vi "Client Monitor.vi"() -> ()   [LabVIEW 2020]
uses:
  source/Client/Subscription/Subscription.lvclass
  source/Value/Value/Value.lvclass
  source/Client/Client/Client.lvclass
  41e1d11c-de9d-40a4-9c04-0640dffbb6fa.vi
panel:
  in  "timeout":dbl[unit]=1.0
  out "Value":dbl
  out "timed out?":bool
  in  "stop":bool
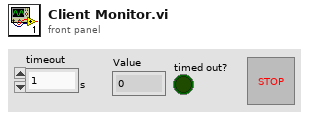
[diagram p1: front panel]
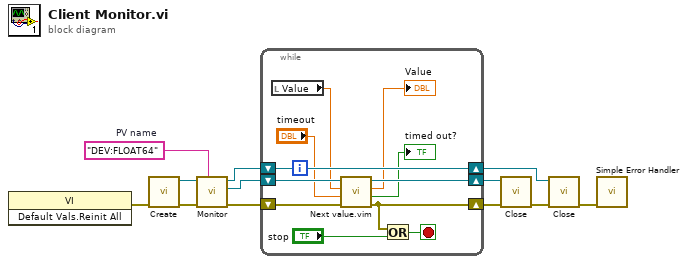
[diagram p0: block diagram]
diagram:
  w6 = "DEV:FLOAT64"  # PV name
  n1 = invoke class="VI" method="Default Vals.Reinit All"() -> (error out=w11:errorcluster)  [unwired: 3 in, 2 out]
  n2 = call "Create.vi"("error in (no error)"=w11) -> ("error out"=w9:errorcluster, "Client out"=w10:refnum<class "Client.lvclass">)  [unwired: 9 in]
  n3 = call "Monitor.vi"("PV name"=w6, "error in"=w9, "Client in"=w10) -> ("error out"=w8:errorcluster, "subscription"=w5:refnum<class "Subscription.lvclass">, "Client out"=w7:refnum<class "Client.lvclass">)  [unwired: 6 in]
  n4 = while {
    shift-right: [w23] -> w12
    shift-left: w7 -> [w23]
    shift-right: [w19] -> w3
    shift-left: w8 -> [w20]
    shift-right: [w17] -> w4
    shift-left: w5 -> [w18]
    stop <- w22 stop-if-true
    n5 = local read "Value"() -> (w15:dbl)
    n6 = call "Next value.vim"("error in"=w20, "timeout"="timeout", "default"=w15, "Subscription in"=w18) -> ("error out"=w19:errorcluster, "timed out?"=→"timed out?":bool, "value"=→"Value":dbl, "Subscription out"=w17:refnum<class "Subscription.lvclass">)  [unwired: 3 in, 1 out]
    n7 = Or(x=w19, y="stop") -> (x .or. y?=w22:bool)
  }
  n8 = call "Close.vi"("error in (no error)"=w3, "Subscription in"=w4) -> ("error out"=w2:errorcluster)  [unwired: 8 in, 1 out]
  n9 = call "Close.vi"("error in (no error)"=w2, "Client in"=w12) -> ("error out"=w1:errorcluster)  [unwired: 9 in]
  n10 = call <vilib>:"Simple Error Handler.vi"("error in (no error)"=w1) -> ()  [unwired: 4 in, 5 out]
